vi "Host.vi"() -> ()   [LabVIEW 2025]
uses:
  <vilib>/FPGAPlugInAG/cRIO-9035/niLvFpga_Open_cRIO-9035.vi
  <vilib>/rvi/interface/common/dynamic/niFpgaDynamicAddResources.vi
  <vilib>/FPGAPlugInAG/Dynamic/niLvFpga_Reset_Dynamic.vi
  <vilib>/Utility/error.llb/Error Cluster From Error Code.vi
  <vilib>/rvi/errors/niLvFpgaAdjustHostInterfaceError.vi
  <vilib>/FPGAPlugInAG/Dynamic/niLvFpga_Run_Dynamic.vi
  <vilib>/FPGAPlugInAG/Dynamic/niLvFpga_Close_Dynamic.vi
  <vilib>/rvi/interface/nirviOpenFPGA/nirviOpenFPGA.xnode
  FPGA Bitfiles/hmmlponfpgav2_FPGATarget_Target_XSyPHY-vVOY.lvbitx
  <vilib>/rvi/interface/nirviMethod/nirviMethod.xnode
  <vilib>/rvi/interface/nirviCloseFPGA/nirviCloseFPGA.xnode
  <vilib>/rvi/errors/niLvFpgaMergeErrorWithErrorCode.vi
  <vilib>/FPGAPlugInAG/Dynamic/niLvFpga_WriteFifo_Dynamic.vi
  <vilib>/FPGAPlugInAG/Dynamic/niLvFpga_ReadFifo_Dynamic.vi
panel:
  out "output array":sgl[](array[numeric])
  out "size(s) 2":i32
  out "Control Force":sgl[](graph)
  out "Window(s)":dbl[][](array[numeric])
  out "Output":sgl[](array[numeric])
  out "input":dbl[][](array[numeric])
  out "size(s)":i32[](array[numeric])
  out "Uncontrolled Acceleration":dynamicdata(graph)
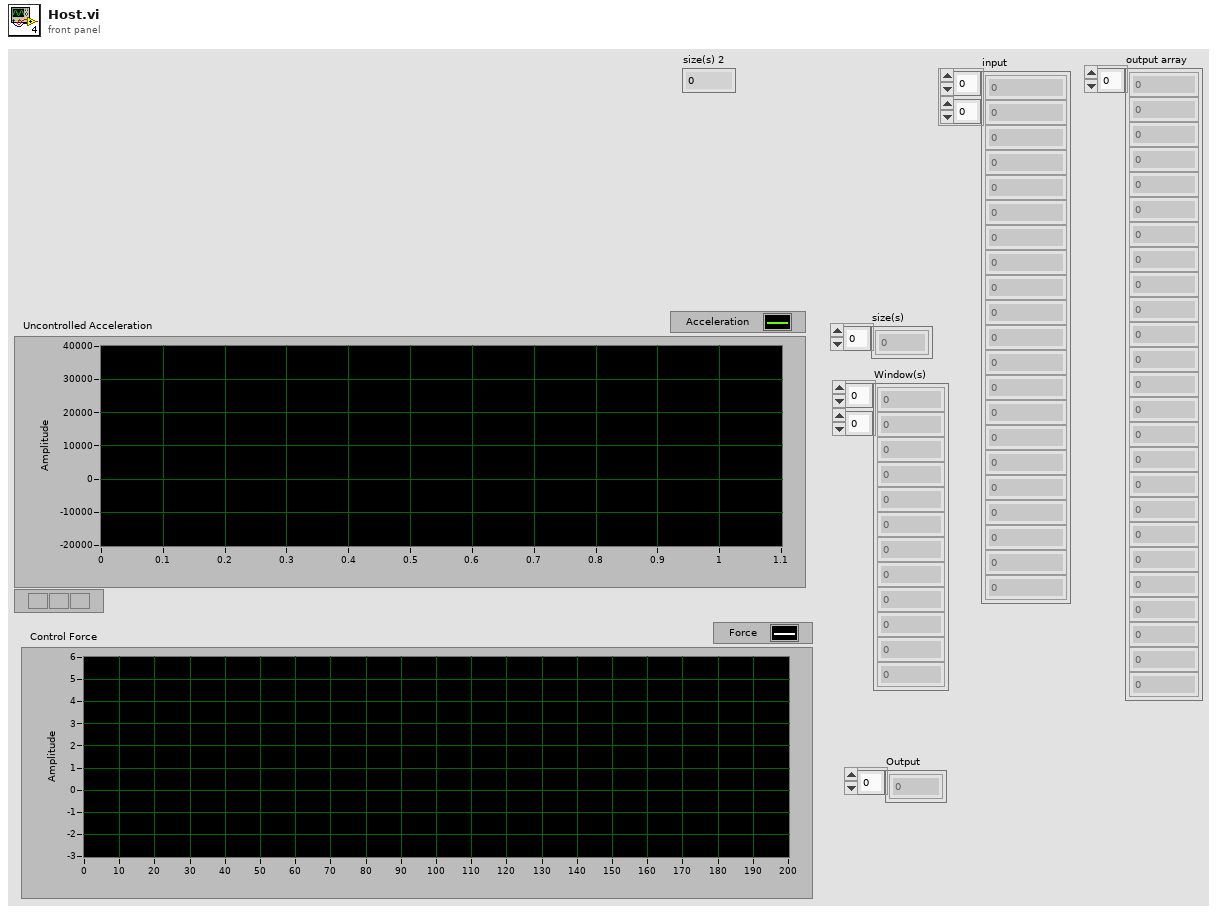
[diagram p1: front panel]
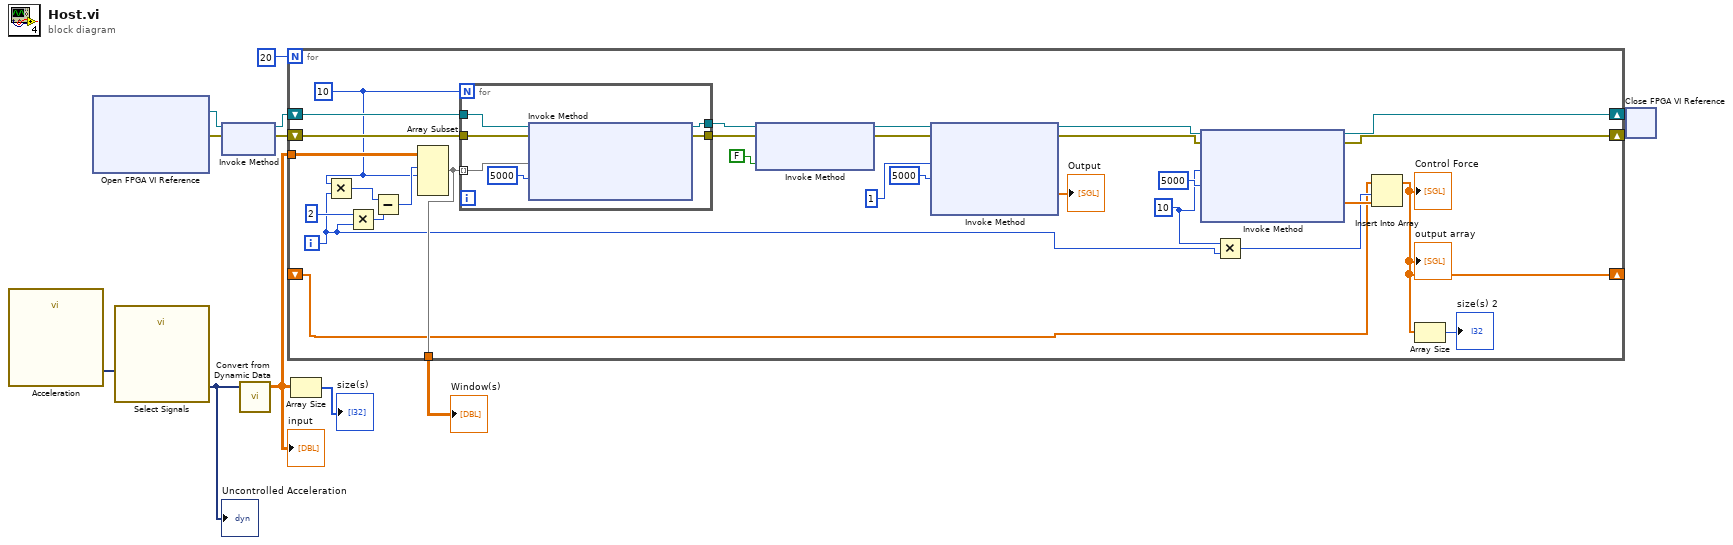
[diagram p0: block diagram]
diagram:
  n1 = call "Acceleration"() -> ("Signals"=w12:dynamicdata)  [unwired: 6 in, 5 out]
  n2 = xnode "Open FPGA VI Reference"() -> ("FPGA VI Reference Out"=w11:refnum<k20>, "error out"=w8:errorcluster)  [unwired: 2 in]
  n3 = call "Select Signals"("Signals"=w12) -> ("Signal Out"=w7:dynamicdata)  [unwired: 9 in, 1 out]
  "Uncontrolled Acceleration" <- w7
  n4 = xnode "Invoke Method"("FPGA VI Reference In"=w11, "error in"=w8) -> ("FPGA VI Reference Out"=w10:refnum<k20>, "error out"=w9:errorcluster)
  n5 = call "Convert from Dynamic Data"("Dynamic Data Type"=w7) -> ("Array"=w2:dbl[][])  [unwired: 3 in]
  "input" <- w2
  n6 = for {
    N: 20 -> [_]
    shift-right: [w17] -> w5
    shift-left: w10 -> [w41]
    shift-right: [w23] -> w4
    shift-left: w9 -> [w40]
    tunnel: w2 -> [w32]
    tunnel: [w30] -> w1
    shift-right: [w22] -> _
    shift-left: _ -> [w19]
    i -> [w15]
    w20 = u32 10 ("Number of Elements")
    w13 = 10
    n7 = Multiply(x=w13, y=w15) -> (x*y=w29:i32)
    n8 = Multiply(x=2 ("y"), y=w15) -> (x*y=w14:i32)
    n9 = Subtract(x=w29, y=w14) -> (x-y=w28:i32)
    n10 = Array Subset(array=w32, index (row)=w28, length (row)=w13) -> (w30:dbl[][])  [unwired: 2 in]
    n11 = for {
      N: w13 -> [_]
      tunnel: w41 -> [w47]
      tunnel: w40 -> [w46]
      tunnel: [w44] -> w36
      tunnel: [w43] -> w35
      tunnel: w30 -> [w42] mode=indexing
      n12 = xnode "Invoke Method"("FPGA VI Reference In"=w47, "error in"=w46, "Data"=w42, "Timeout (ms)"=5000) -> ("FPGA VI Reference Out"=w44:refnum<k20>, "error out"=w43:errorcluster)  [unwired: 1 out]
    }
    n13 = xnode "Invoke Method"("FPGA VI Reference In"=w36, "error in"=w35, "Wait Until Done (F)"=FALSE) -> ("FPGA VI Reference Out"=w38:refnum<k20>, "error out"=w37:errorcluster)
    n14 = xnode "Invoke Method"("FPGA VI Reference In"=w38, "error in"=w37, "Number of Elements"=u32 1, "Timeout (ms)"=5000) -> ("FPGA VI Reference Out"=w18:refnum<k20>, "error out"=w24:errorcluster, "Data"=→"Output":sgl[])  [unwired: 1 out]
    n15 = xnode "Invoke Method"("FPGA VI Reference In"=w18, "error in"=w24, "Number of Elements"=w20, "Timeout (ms)"=5000) -> ("FPGA VI Reference Out"=w17:refnum<k20>, "error out"=w23:errorcluster, "Data"=w26:sgl[])  [unwired: 1 out]
    n16 = Multiply(x=w20, y=w15) -> (x*y=w25:u32)
    n17 = Insert Into Array(array=w19, index=w25, new element=w26) -> (w22:sgl[])
    "Control Force" <- w22
    "output array" <- w22
    n18 = Array Size(array=w22) -> (size(s)=→"size(s) 2":i32)
  }
  "Window(s)" <- w1
  n19 = Array Size(array=w2) -> (size(s)=→"size(s)":i32[])
  n20 = xnode "Close FPGA VI Reference"("FPGA VI Reference In"=w5, "error in"=w4) -> ()  [unwired: 1 out]
